vi "VFD motor control.vi"(0 "MotorQueue":refnum<queue>, 4 "Stop-Pump":bool, 5 "Start Pump":bool, 7 "Start Motor":bool, 8 "Pump speed (%)":dbl=1.0 min=1.0 max=99.0, 10 "Control Cluster":T1, 11 "Stop all":bool) -> ()   [LabVIEW 2021]
panel:
  in  "Stop-Motor":bool
  in  "Motor speed (%)":dbl=1.0 min=1.0 max=70.0
  in  "DigitalQueue":refnum<queue>
  in  "Set Motor Brake":bool
  in  "Enable Motor":bool
  in  "Sequence to run on start up 3":string[](array[string])=[""]
  out "Motor System State":string="Idle"
  in  "Enable Motor/Pumps\nControl Board":bool
  in  "Set Digital Lines":bool
  out "Pump System State":string="Idle"
  in  "Sequence to run on start up 2":string[](array[string])=[""]
  in  "PWM Frequency [Hz]":dbl=10000.0
  out "Digital system state":string="Idle"
  in  "Sequence to run on start up":string[](array[string])=[""]
  # "Speed indicators"
  # "When the green button is on (lit) \nfor the brake and clutch, \nthey are disconnected"
  # "For the Motor Enable and Direction, when\nthe green button is on, they are connected/enabled"
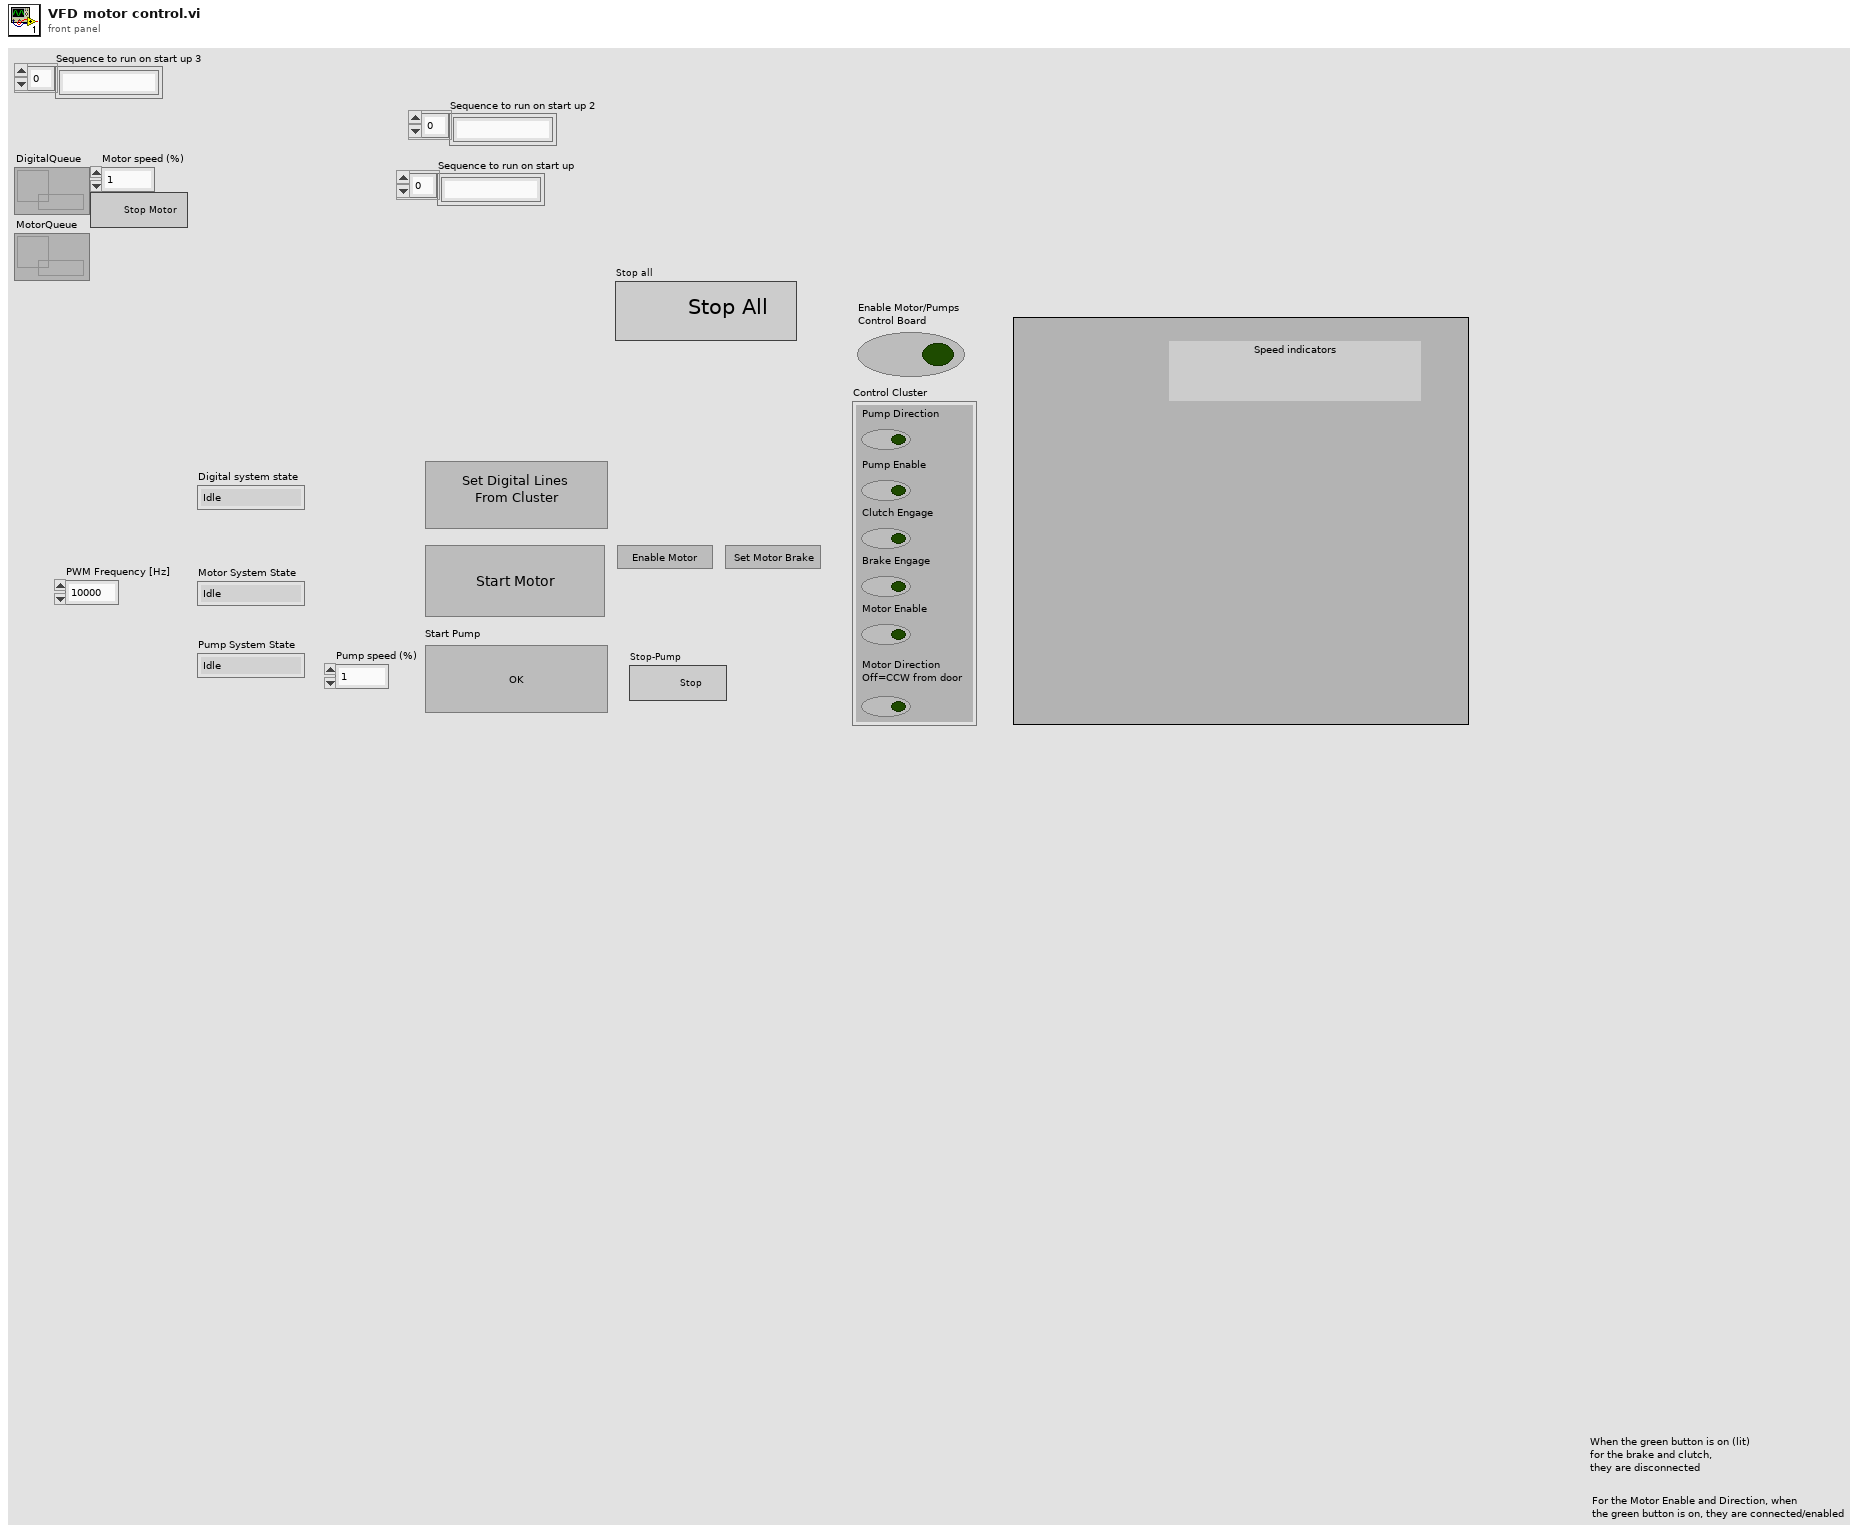
[diagram p1: front panel]
types:
  T1 = cluster{"Pump Direction":bool, "Pump Enable":bool, "Clutch Engage":bool, "Brake Engage":bool, "Motor Enable":bool, "Motor Direction\nOff=CCW from door":bool}
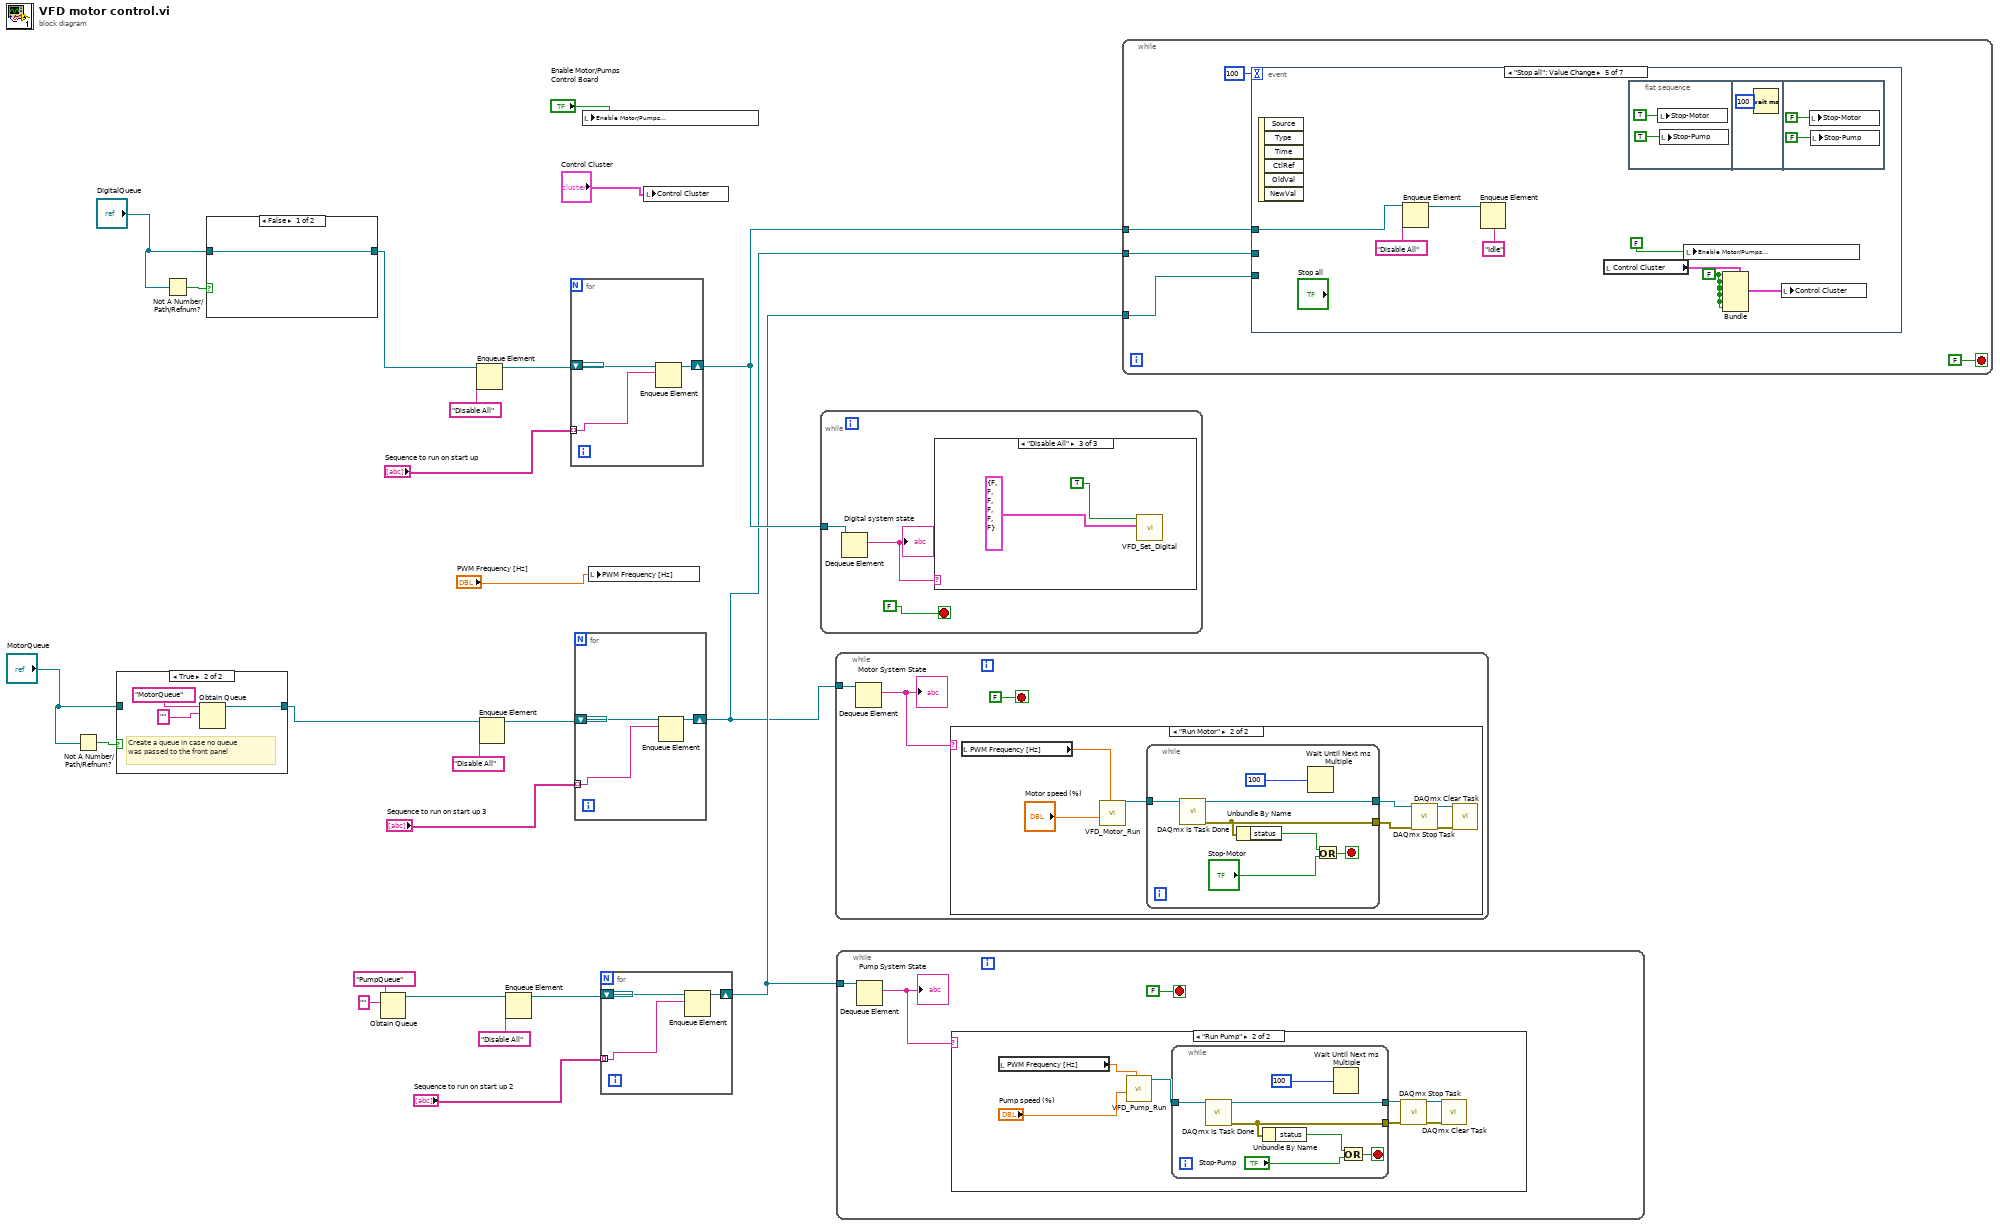
[diagram p0: block diagram]
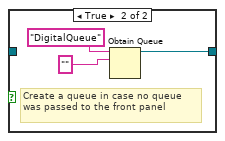
[diagram p3: hidden frame]
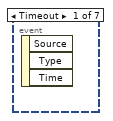
[diagram p6: hidden frame]
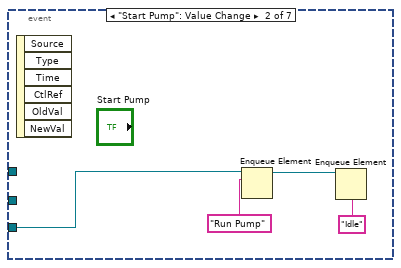
[diagram p7: hidden frame]
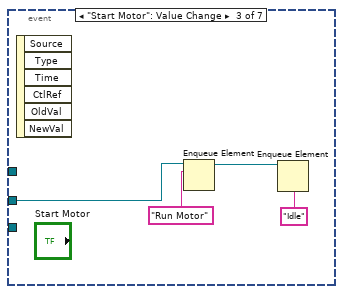
[diagram p8: hidden frame]
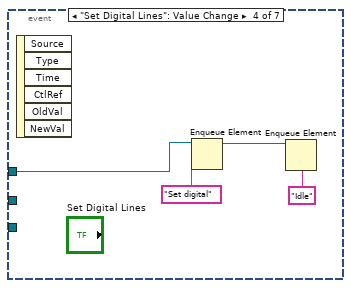
[diagram p9: hidden frame]
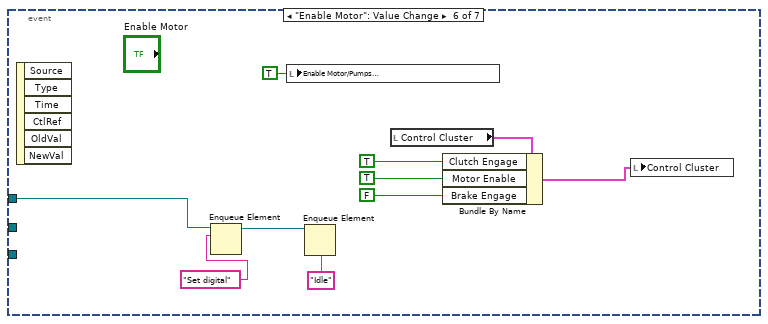
[diagram p10: hidden frame]
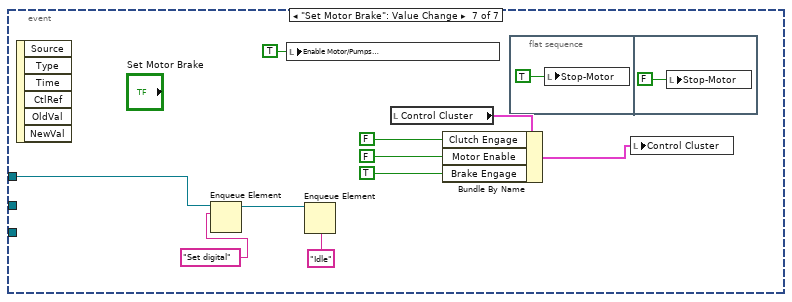
[diagram p11: hidden frame]
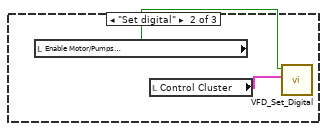
[diagram p13: hidden frame]
diagram:
  n1 = Not A Number/Path/Refnum?(number/path/refnum="MotorQueue") -> (NaN/Path/Refnum?=w2:bool)
  n2 = case shown="True" w2 {
    tunnel: "MotorQueue" -> [w25 _]
    tunnel: [w25 w28] -> w1
    frame False {
    }
    frame True {
      # "Create a queue in case no queue was passed to the front panel"
      n3 = Obtain Queue(name (unnamed)="MotorQueue", element data type="" ("Type def")) -> (queue out=w28:refnum<queue>)  [unwired: 3 in, 2 out]
    }
  }
  n4 = Not A Number/Path/Refnum?(number/path/refnum="DigitalQueue") -> (NaN/Path/Refnum?=w6:bool)
  n5 = case shown="False" w6 {
    tunnel: "DigitalQueue" -> [w29 _]
    tunnel: [w29 w32] -> w4
    frame False {
    }
    frame True {
      # "Create a queue in case no queue was passed to the front panel"
      n6 = Obtain Queue(name (unnamed)="DigitalQueue", element data type="" ("Type def")) -> (queue out=w32:refnum<queue>)  [unwired: 3 in, 2 out]
    }
  }
  n7 = Obtain Queue(name (unnamed)="PumpQueue", element data type="" ("Type def")) -> (queue out=w17:refnum<queue>)  [unwired: 3 in, 2 out]
  n8 = Enqueue Element(queue=w4, element="Disable All") -> (queue out=w23:refnum<queue>)  [unwired: 2 in, 2 out]
  n9 = Enqueue Element(queue=w1, element="Disable All") -> (queue out=w9:refnum<queue>)  [unwired: 2 in, 2 out]
  n10 = Enqueue Element(queue=w17, element="Disable All") -> (queue out=w18:refnum<queue>)  [unwired: 2 in, 2 out]
  n11 = for {
    shift-right: [w33] -> w21
    shift-left: w23 -> [w34]
    tunnel: "Sequence to run on start up" -> [w35] mode=indexing
    n12 = Enqueue Element(queue=w34, element=w35) -> (queue out=w33:refnum<queue>)  [unwired: 2 in, 2 out]
  }
  n13 = for {
    shift-right: [w36] -> w7
    shift-left: w9 -> [w37]
    tunnel: "Sequence to run on start up 3" -> [w38] mode=indexing
    n14 = Enqueue Element(queue=w37, element=w38) -> (queue out=w36:refnum<queue>)  [unwired: 2 in, 2 out]
  }
  n15 = local write "Enable Motor/Pumps\nControl Board"("Enable Motor/Pumps\nControl Board") -> ()
  n16 = local write "PWM Frequency [Hz]"("PWM Frequency [Hz]") -> ()
  n17 = for {
    shift-right: [w39] -> w13
    shift-left: w18 -> [w40]
    tunnel: "Sequence to run on start up 2" -> [w41] mode=indexing
    n18 = Enqueue Element(queue=w40, element=w41) -> (queue out=w39:refnum<queue>)  [unwired: 2 in, 2 out]
  }
  n19 = local write "Control Cluster"("Control Cluster") -> ()
  n20 = while {
    tunnel: w21 -> [w44]
    stop <- FALSE stop-if-true
    n21 = Dequeue Element(queue=w44) -> (element=w43:string)  [unwired: 2 in, 3 out]
    "Digital system state" <- w43
    n22 = case shown="\"Disable All\"" w43 {
      frame "Idle", Default {
      }
      frame "Set digital" {
        n23 = local read "Enable Motor/Pumps\nControl Board"() -> (w46:bool)
        n24 = local read "Control Cluster"() -> (w45:T1)
        n25 = call "VFD_Set_Digital.vi"("Control Cluster"=w45, "Enable Motor/Pumps\nControl Board"=w46) -> ()  [unwired: 10 in]
      }
      frame "Disable All" {
        n26 = call "VFD_Set_Digital.vi"("Control Cluster"=T1 {"Pump Direction"=FALSE, "Pump Enable"=FALSE, "Clutch Engage"=FALSE, "Brake Engage"=FALSE, "Motor Enable"=FALSE, "Motor Direction\nOff=CCW from door"=FALSE} ("Control Cluster 2"), "Enable Motor/Pumps\nControl Board"=TRUE) -> ()  [unwired: 10 in]
      }
    }
  }
  n27 = while {
    tunnel: w7 -> [w49]
    stop <- FALSE stop-if-true
    n28 = Dequeue Element(queue=w49) -> (element=w50:string)  [unwired: 2 in, 3 out]
    "Motor System State" <- w50
    n29 = case shown="\"Run Motor\"" w50 {
      frame "Idle", Default {
      }
      frame "Run Motor" {
        n30 = local read "PWM Frequency [Hz]"() -> (w57:dbl)
        n31 = call "VFD_Motor_Run.vi"("PWM Frequency [Hz]"=w57, "Motor speed (%)"="Motor speed (%)") -> ("task out"=w52:refnum<k21>)  [unwired: 9 in]
        n32 = while {
          tunnel: w52 -> [w65]
          tunnel: [w62] -> w55
          tunnel: [w63] -> w54
          stop <- w64 stop-if-true
          n33 = call <vilib>:"DAQmx Is Task Done.vi"("task/channels in"=w65) -> ("task out"=w63:refnum<k21>, "error out"=w62:errorcluster)  [unwired: 12 in, 1 out]
          n34 = Unbundle By Name(w62) -> ("status"=w61:bool)
          n35 = Wait Until Next ms Multiple(millisecond multiple=u32 100) -> ()  [unwired: 1 out]
          n36 = Or(x=w61, y="Stop-Motor") -> (x .or. y?=w64:bool)
        }
        n37 = call <vilib>:"DAQmx Stop Task.vi"("task/channels in"=w54, "error in"=w55) -> ("task out"=w53:refnum<k21>, "error out"=w56:errorcluster)  [unwired: 12 in]
        n38 = call <vilib>:"DAQmx Clear Task.vi"("task in"=w53, "error in"=w56) -> ()  [unwired: 13 in, 1 out]
      }
    }
  }
  n39 = while {
    tunnel: w13 -> [w66]
    stop <- FALSE stop-if-true
    n40 = Dequeue Element(queue=w66) -> (element=w67:string)  [unwired: 2 in, 3 out]
    "Pump System State" <- w67
    n41 = case shown="\"Run Pump\"" w67 {
      frame "Idle", Default {
      }
      frame "Run Pump" {
        n42 = local read "PWM Frequency [Hz]"() -> (w75:dbl)
        n43 = call "VFD_Pump_Run.vi"("PWM Frequency [Hz]"=w75, "Pump speed (%)"="Pump speed (%)") -> ("task out"=w69:refnum<k21>)  [unwired: 9 in]
        n44 = while {
          tunnel: [w80] -> w70
          tunnel: [w81] -> w71
          tunnel: w69 -> [w77]
          stop <- w82 stop-if-true
          n45 = call <vilib>:"DAQmx Is Task Done.vi"("task/channels in"=w77) -> ("task out"=w81:refnum<k21>, "error out"=w80:errorcluster)  [unwired: 12 in, 1 out]
          n46 = Unbundle By Name(w80) -> ("status"=w79:bool)
          n47 = Wait Until Next ms Multiple(millisecond multiple=u32 100) -> ()  [unwired: 1 out]
          n48 = Or(x=w79, y="Stop-Pump") -> (x .or. y?=w82:bool)
        }
        n49 = call <vilib>:"DAQmx Stop Task.vi"("task/channels in"=w71, "error in"=w70) -> ("task out"=w73:refnum<k21>, "error out"=w72:errorcluster)  [unwired: 12 in]
        n50 = call <vilib>:"DAQmx Clear Task.vi"("task in"=w73, "error in"=w72) -> ()  [unwired: 13 in, 1 out]
      }
    }
  }
  n51 = while {
    tunnel: w21 -> [w87]
    tunnel: w13 -> [w85]
    tunnel: w7 -> [w84]
    stop <- FALSE stop-if-true
    n52 = event shown="[4] \"Stop all\": Value Change" {
      selector: _ -> [_ _ _ _ _ _ _]
      dyn-events: _ -> [_ _ _ _ _ _ _]
      timeout: 100 -> [_ _ _ _ _ _ _]
      tunnel: w87 -> [_ _ _ w96 w104 w115 w125]
      tunnel: w85 -> [_ w88 _ _ _ _ _]
      tunnel: w84 -> [_ _ w92 _ _ _ _]
      event Timeout {
        n53 = event-data() -> ()  [unwired: 1 in, 3 out]
      }
      event "Start Pump": Value Change {
        n54 = event-data() -> ()  [unwired: 1 in, 6 out]
        n55 = Enqueue Element(queue=w88, element="Run Pump") -> (queue out=w89:refnum<queue>)  [unwired: 2 in, 2 out]
        n56 = Enqueue Element(queue=w89, element="Idle") -> ()  [unwired: 2 in, 3 out]
      }
      event "Start Motor": Value Change {
        n57 = event-data() -> ()  [unwired: 1 in, 6 out]
        n58 = Enqueue Element(queue=w92, element="Run Motor") -> (queue out=w93:refnum<queue>)  [unwired: 2 in, 2 out]
        n59 = Enqueue Element(queue=w93, element="Idle") -> ()  [unwired: 2 in, 3 out]
      }
      event "Set Digital Lines": Value Change {
        n60 = event-data() -> ()  [unwired: 1 in, 6 out]
        n61 = Enqueue Element(queue=w96, element="Set digital") -> (queue out=w97:refnum<queue>)  [unwired: 2 in, 2 out]
        n62 = Enqueue Element(queue=w97, element="Idle") -> ()  [unwired: 2 in, 3 out]
      }
      event "Stop all": Value Change {
        w102 = FALSE ("Pump Direction")
        n63 = event-data() -> ()  [unwired: 1 in, 6 out]
        n64 = Enqueue Element(queue=w104, element="Disable All") -> (queue out=w105:refnum<queue>)  [unwired: 2 in, 2 out]
        n65 = Enqueue Element(queue=w105, element="Idle") -> ()  [unwired: 2 in, 3 out]
        n66 = local read "Control Cluster"() -> (w103:T1)
        n67 = flat-sequence {
          frame #0 {
            n68 = local write "Stop-Motor"(TRUE ("Stop-Motor")) -> ()
            n69 = local write "Stop-Pump"(TRUE ("Stop-Motor")) -> ()
          }
          frame #1 {
            n70 = Wait (ms)(milliseconds to wait=u32 100) -> ()  [unwired: 1 out]
          }
          frame #2 {
            n71 = local write "Stop-Motor"(FALSE ("Stop-Motor")) -> ()
            n72 = local write "Stop-Pump"(FALSE ("Stop-Motor")) -> ()
          }
        }
        n73 = local write "Enable Motor/Pumps\nControl Board"(FALSE ("Enable Motor/Pumps")) -> ()
        n74 = Bundle(cluster=w103, "Pump Direction"=w102, "Pump Enable"=w102, "Clutch Engage"=w102, "Brake Engage"=w102, "Motor Enable"=w102, "Motor Direction\nOff=CCW from door"=w102) -> (w101:T1)
        n75 = local write "Control Cluster"(w101) -> ()
      }
      event "Enable Motor": Value Change {
        n76 = event-data() -> ()  [unwired: 1 in, 6 out]
        n77 = Enqueue Element(queue=w115, element="Set digital") -> (queue out=w116:refnum<queue>)  [unwired: 2 in, 2 out]
        n78 = local write "Enable Motor/Pumps\nControl Board"(TRUE ("Enable Motor/Pumps\nControl Board")) -> ()
        n79 = Enqueue Element(queue=w116, element="Idle") -> ()  [unwired: 2 in, 3 out]
        n80 = local read "Control Cluster"() -> (w122:T1)
        n81 = Bundle By Name(cluster=w122, "Clutch Engage"=TRUE, "Motor Enable"=TRUE, "Brake Engage"=FALSE ("Motor Direction\nOff=CCW from door")) -> (w121:T1)
        n82 = local write "Control Cluster"(w121) -> ()
      }
      event "Set Motor Brake": Value Change {
        n83 = event-data() -> ()  [unwired: 1 in, 6 out]
        n84 = Enqueue Element(queue=w125, element="Set digital") -> (queue out=w126:refnum<queue>)  [unwired: 2 in, 2 out]
        n85 = local write "Enable Motor/Pumps\nControl Board"(TRUE ("Enable Motor/Pumps\nControl Board")) -> ()
        n86 = Enqueue Element(queue=w126, element="Idle") -> ()  [unwired: 2 in, 3 out]
        n87 = local read "Control Cluster"() -> (w132:T1)
        n88 = Bundle By Name(cluster=w132, "Clutch Engage"=FALSE, "Motor Enable"=FALSE, "Brake Engage"=TRUE ("Motor Direction\nOff=CCW from door")) -> (w131:T1)
        n89 = flat-sequence {
          frame #0 {
            n90 = local write "Stop-Motor"(TRUE ("Stop-Motor")) -> ()
          }
          frame #1 {
            n91 = local write "Stop-Motor"(FALSE ("Stop-Motor")) -> ()
          }
        }
        n92 = local write "Control Cluster"(w131) -> ()
      }
    }
  }
